vi "Destroy.vi"(0 "reference in":refnum<class "LoggerAdapter.lvclass">, 11 "Error In":errorcluster) -> (4 "reference out":refnum<class "LoggerAdapter.lvclass">, 15 "Error Out":errorcluster)   [LabVIEW 2024, in "LoggerAdapter.lvclass"]
uses:
  LoggerAdapter.lvclass
  Logger_class/Logger.lvclass
  LoggerAdapter.lvclass/LoggerAdapter.ctl
panel:
  # "Connector Pane"
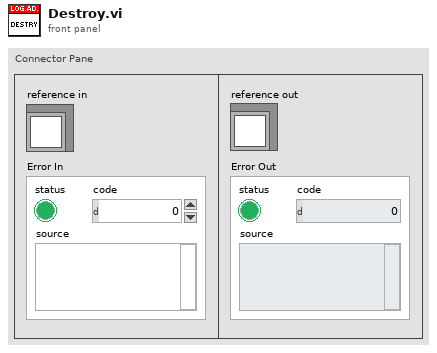
[diagram p1: front panel]
types:
  T1 = typedef "LoggerAdapter.lvclass/ObjectAttributes.ctl" = cluster{"Adaptee":refnum<class "Logger.lvclass">}
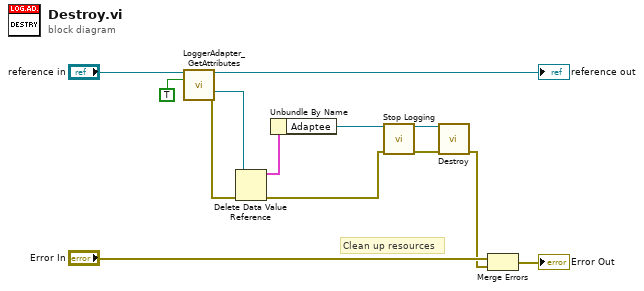
[diagram p0: block diagram]
diagram:
  # "Clean up resources"
  n1 = call "LoggerAdapter_GetAttributes.vi"("reference in"="reference in", "OnlyGetDvrReference(False)"=TRUE) -> ("reference out"=→"reference out":refnum<class "LoggerAdapter.lvclass">, "DataRef"=w9:refnum<data-value>, "Error Out"=w10:errorcluster)  [unwired: 10 in, 1 out]
  n2 = Delete Data Value Reference(data value reference=w9, error in=w10) -> (data value=w6:T1, error out=w5:errorcluster)
  n3 = Unbundle By Name(w6) -> ("Adaptee"=w2:refnum<class "Logger.lvclass">)
  n4 = call-dynamic "Stop Logging.vi"("reference in"=w2, "Error In"=w5) -> ("reference out"=w1:refnum<class "Logger.lvclass">, "Error Out"=w3:errorcluster)  [unwired: 12 in]
  n5 = call-dynamic "Destroy.vi"("reference in"=w1, "Error In"=w3) -> ("Error Out"=w4:errorcluster)  [unwired: 12 in, 1 out]
  n6 = Merge Errors("Error In", w4) -> (→"Error Out":errorcluster)
